vi "run.get.multiple.vi"(8 "error in":errorcluster, 10 "rid(s)":string[](array[string]), 11 "Nominal Client in":refnum<class "Nominal Client.lvclass">) -> (0 "error out":errorcluster, 2 "Runs":refnum<class "Run.lvclass">[](array[class]), 3 "Nominal Client out":refnum<class "Nominal Client.lvclass">, 4 "Response body":string)   [LabVIEW 2020, in "Nominal Client.lvclass"]
doc: "Fetches details about the run in question based on its RID."
uses:
  Nominal Client.lvclass
  Run/Run.lvclass
  49411445-db77-4211-b7bb-06afe579b778.vi
  <vilib>/JDP Science/JSONtext/Variant to JSON Text.vi
  <vilib>/JDP Science/JSONtext/LVClass Serializer/JSONtext LVClass Serializer.lvclass
  Nominal Client.lvclass/Nominal Client.ctl
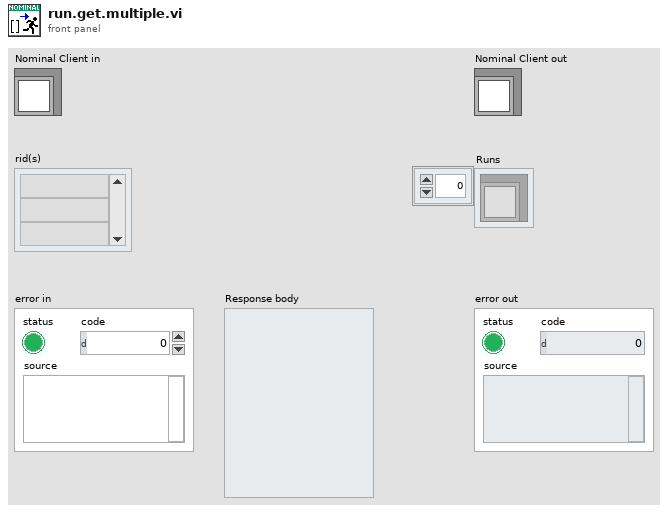
[diagram p1: front panel]
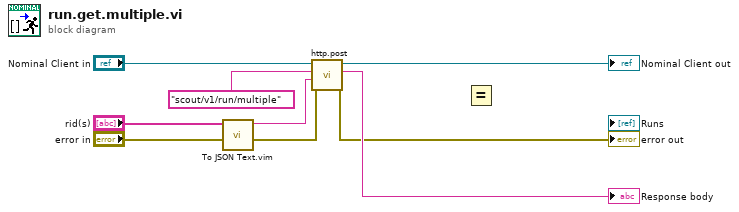
[diagram p0: block diagram]
diagram:
  n1 = call "To JSON Text.vim"("error in (no error)"="error in", "Anything"="rid(s)") -> ("error out"=w3:errorcluster, "<JSON>"=w2:string)  [unwired: 8 in]
  n2 = call "http.post.vi"("error in"=w3, "Request body"=w2, "Path"="scout/v1/run/multiple", "Nominal Client in"="Nominal Client in") -> ("error out"=→"error out":errorcluster, "Response"=→"Response body":string, "Nominal Client out"=→"Nominal Client out":refnum<class "Nominal Client.lvclass">)  [unwired: 4 in, 1 out]
  n3 = Equal?() -> ()  [unwired: 2 in, 1 out]
